vi "SelectCycle.vi"   [LabVIEW 2019]
uses:
  02 Mode/SerialMode/SerialClass.lvclass
  02 Mode/TCPClientMode/TCPClientClass.lvclass
  02 Mode/TCPServerMode/TCPServerClass.lvclass
panel:
  # "带有发送的功能不能和单侦听的挤在一个循环内\n否则会导致时间强行同步，未选中的也要等待发送侦听完成\n\n且对于串口自发自收的情况，由于强制循环同步导致发送方无法准确获取反馈\n因为反馈方在等待状态，完成后才能收到命令再反馈，但是发送方已超时"
types:
  T1 = cluster{"串口名":string, "串口类":refnum<class "SerialClass.lvclass">}
  T2 = typedef "串口枚举.ctl" = enum16{"ini", "增", "删", "查", "改"}
  T3 = cluster{"客服名":string, "客服类":refnum<class "TCPClientClass.lvclass">}
  T4 = cluster{"没有记录？":bool, "串口类":refnum<class "SerialClass.lvclass">}
  T5 = typedef "SerialData.ctl" = cluster{"VISA串口名称":refnum<visa-resource-name>, "波特率":u32, "停止位":u16, "流控制":u16, "数据位":u16, "奇偶校验":enum16{"None", "Odd", "Even", "Mark", "Space"}, "超时":u32, "启用终止符？":bool, "终止符":u8}
  T6 = cluster{"未找到?":bool, "客服类":refnum<class "TCPClientClass.lvclass">}
  T7 = map{string, refnum<class "TCPServerClass.lvclass">}
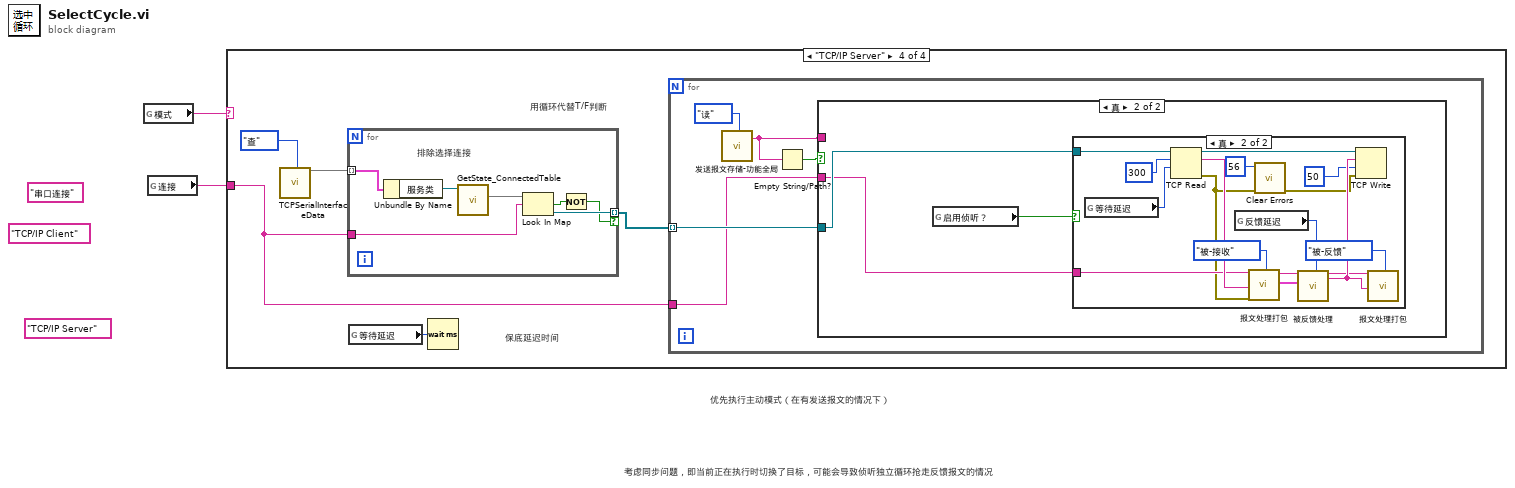
[diagram p0: block diagram]
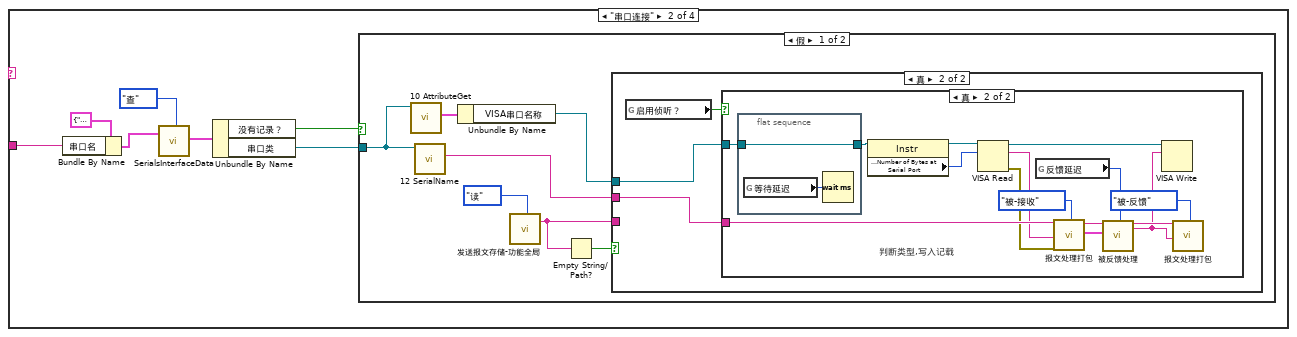
[diagram p3: hidden frame]
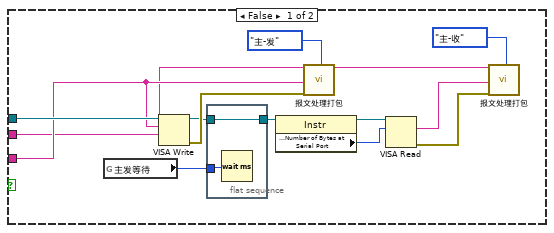
[diagram p4: hidden frame]
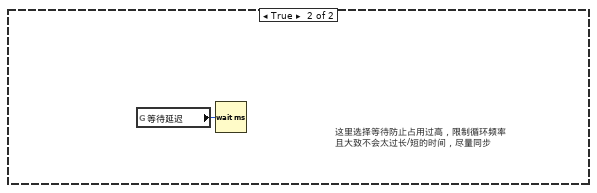
[diagram p6: hidden frame]
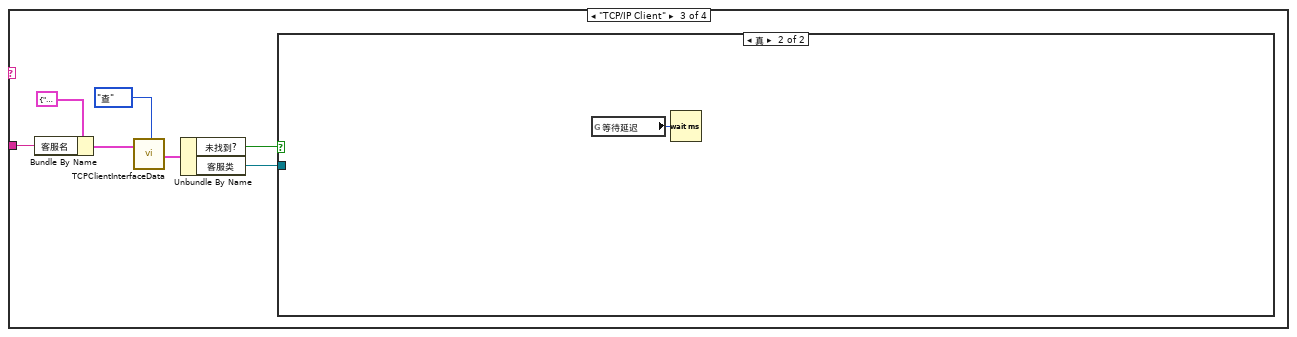
[diagram p7: hidden frame]
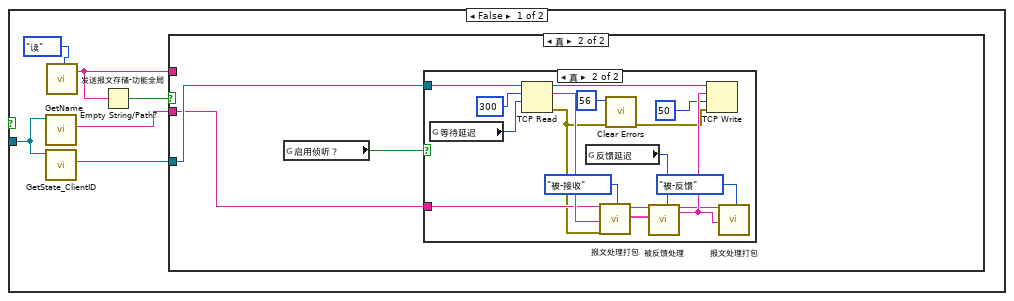
[diagram p8: hidden frame]
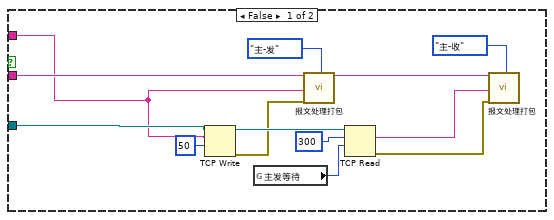
[diagram p9: hidden frame]
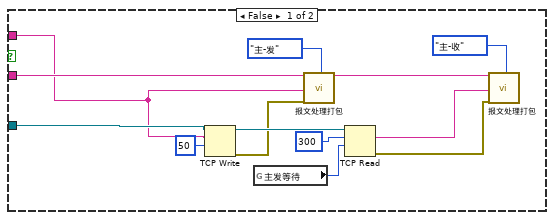
[diagram p11: hidden frame]
diagram:
  (unwired) "TCP/IP Server" ("y")
  (unwired) "TCP/IP Client" ("y")
  (unwired) "串口连接" ("y")
  # "考虑同步问题，即当前正在执行时切换了目标，可能会导致侦听独立循环抢走反馈报文的情况"
  # "优先执行主动模式（在有发送报文的情况下）"
  n1 = global read "全局-配置识别.vi" "模式"() -> (w2:string)
  n2 = global read "全局-配置识别.vi" "连接"() -> (w1:string)
  n3 = case shown="\"TCP/IP Server\"" w2 {
    tunnel: w1 -> [_ w3 w59 w102]
    frame "假", Default {
    }
    frame "串口连接" {
      n4 = Bundle By Name(cluster=T1 {"串口名"="", "串口类"=refnum} ("信息"), "串口名"=w3) -> (w7:T1)
      n5 = call "SerialsInterfaceData.vi"("信息"=w7, "串口枚举"=串口枚举."查") -> ("查找结果"=w6:T4)  [unwired: 16 in, 1 out]
      n6 = Unbundle By Name(w6) -> ("没有记录？"=w5:bool, "串口类"=w4:refnum<class "SerialClass.lvclass">)
      n7 = case shown="假" w5 {
        tunnel: w4 -> [w15 _]
        frame False {
          n8 = call-dynamic "10 AttributeGet.vi"("SerialClass 输入"=w15) -> ("串口配置"=w16:T5)  [unwired: 7 in, 3 out]
          n9 = call-dynamic "12 SerialName.vi"("SerialClass 输入"=w15) -> ("串口名称"=w11:string)  [unwired: 8 in, 2 out]
          n10 = Unbundle By Name(w16) -> ("VISA串口名称"=w10:refnum<visa-resource-name>)
          n11 = call "发送报文存储-功能全局.vi"("枚举"=enum16{"ini", "读", "写"}."读") -> ("报文输出"=w14:string)  [unwired: 18 in]
          n12 = Empty String/Path?(string/path=w14) -> (empty?=w13:bool)
          n13 = case shown="真" w13 {
            tunnel: w10 -> [w28 w34]
            tunnel: w14 -> [w23 _]
            tunnel: w11 -> [w17 w33]
            frame False {
              n14 = global read "全局-配置识别.vi" "主发等待"() -> (w18:u32)
              n15 = VISA Write(VISA resource name=w28, write buffer=w23) -> (VISA resource name out=w20:refnum<visa-resource-name>, error out=w21:errorcluster)  [unwired: 1 in, 1 out]
              n16 = flat-sequence {
                tunnel: w20 -> [w32]
                tunnel: [w32] -> w19
                tunnel: w18 -> [w31]
                frame #0 {
                  n17 = Wait (ms)(milliseconds to wait=w31) -> ()  [unwired: 1 out]
                }
              }
              n18 = property class="Instr"(reference=w19) -> (reference out=w29:refnum<visa-resource-name>, "Serial Settings:Number of Bytes at Serial Port"=w30:u32)  [unwired: 1 in, 1 out]
              n19 = call "报文处理打包.vi"("识别名称"=w17, "报文"=w23, "Error In"=w21, "类型"=enum16{"被-接收", "被-反馈", "主-发", "主-收"}."主-发") -> ("识别名称输出"=w24:string)  [unwired: 14 in, 1 out]
              n20 = VISA Read(VISA resource name=w29, byte count=w30) -> (read buffer=w25:string, error out=w22:errorcluster)  [unwired: 1 in, 2 out]
              n21 = call "报文处理打包.vi"("识别名称"=w24, "报文"=w25, "Error In"=w22, "类型"=enum16{"被-接收", "被-反馈", "主-发", "主-收"}."主-收") -> ()  [unwired: 14 in, 2 out]
            }
            frame True {
              n22 = global read "全局-被反馈配置.vi" "启用侦听？"() -> (w35:bool)
              n23 = case shown="真" w35 {
                tunnel: w34 -> [_ w36]
                tunnel: w33 -> [_ w48]
                frame False {
                }
                frame True {
                  # "判断类型,写入记载"
                  n24 = flat-sequence {
                    tunnel: [w52] -> w37
                    tunnel: w36 -> [w52]
                    frame #0 {
                      n25 = global read "全局-配置识别.vi" "等待延迟"() -> (w51:u32)
                      n26 = Wait (ms)(milliseconds to wait=w51) -> ()  [unwired: 1 out]
                    }
                  }
                  n27 = property class="Instr"(reference=w37) -> (reference out=w50:refnum<visa-resource-name>, "Serial Settings:Number of Bytes at Serial Port"=w49:u32)  [unwired: 1 in, 1 out]
                  n28 = VISA Read(VISA resource name=w50, byte count=w49) -> (VISA resource name out=w45:refnum<visa-resource-name>, read buffer=w47:string, error out=w44:errorcluster)  [unwired: 1 in, 1 out]
                  n29 = global read "全局-配置识别.vi" "反馈延迟"() -> (w38:u32)
                  n30 = call "报文处理打包.vi"("识别名称"=w48, "报文"=w47, "Error In"=w44, "类型"=enum16{"被-接收", "被-反馈", "主-发", "主-收"}."被-接收") -> ("识别名称输出"=w43:string, "被收校验信息"=w42:cluster{"可用？":bool, "功能码":u8, "无crc报文":u8[]})  [unwired: 14 in]
                  n31 = call "被反馈处理.vi"("识别名称"=w43, "校验信息"=w42, "等待时间（毫秒）"=w38) -> ("识别名称输出"=w41:string, "反馈"=w40:string)  [unwired: 15 in]
                  n32 = VISA Write(VISA resource name=w45, write buffer=w40) -> ()  [unwired: 1 in, 3 out]
                  n33 = call "报文处理打包.vi"("识别名称"=w41, "报文"=w40, "类型"=enum16{"被-接收", "被-反馈", "主-发", "主-收"}."被-反馈") -> ()  [unwired: 15 in, 2 out]
                }
              }
            }
          }
        }
        frame True {
          # "这里选择等待防止占用过高，限制循环频率\n且大致不会太过长/短的时间，尽量同步"
          n34 = global read "全局-配置识别.vi" "等待延迟"() -> (w53:u32)
          n35 = Wait (ms)(milliseconds to wait=w53) -> ()  [unwired: 1 out]
        }
      }
    }
    frame "TCP/IP Client" {
      n36 = Bundle By Name(cluster=T3 {"客服名"="", "客服类"=refnum} ("信息"), "客服名"=w59) -> (w58:T3)
      n37 = call "TCPClientInterfaceData.vi"("信息"=w58, "客服接口枚举"=enum16{"ini", "增", "删", "查", "改"}."查") -> ("查找结果"=w56:T6)  [unwired: 16 in, 1 out]
      n38 = Unbundle By Name(w56) -> ("未找到?"=w55:bool, "客服类"=w54:refnum<class "TCPClientClass.lvclass">)
      n39 = case shown="真" w55 {
        tunnel: w54 -> [w62 _]
        frame False {
          n40 = call-dynamic "GetName.vi"("TCPClientClass 输入"=w62) -> ("结果字符串"=w61:string)  [unwired: 8 in, 2 out]
          n41 = call-dynamic "GetState_ClientID.vi"("TCPClientClass输入"=w62) -> ("连接ID"=w63:refnum<k5>)  [unwired: 8 in, 2 out]
          n42 = call "发送报文存储-功能全局.vi"("枚举"=enum16{"ini", "读", "写"}."读") -> ("报文输出"=w66:string)  [unwired: 18 in]
          n43 = Empty String/Path?(string/path=w66) -> (empty?=w65:bool)
          n44 = case shown="真" w65 {
            tunnel: w63 -> [w79 w81]
            tunnel: w66 -> [w74 _]
            tunnel: w61 -> [w75 w80]
            frame False {
              n45 = TCP Write(connection ID=w79, data in=w74, 9:50 ("超时毫秒(25000)")) -> (connection ID out=w72:refnum<k5>, error out=w71:errorcluster)  [unwired: 1 in, 1 out]
              n46 = global read "全局-配置识别.vi" "主发等待"() -> (w70:u32)
              n47 = call "报文处理打包.vi"("识别名称"=w75, "报文"=w74, "Error In"=w71, "类型"=enum16{"被-接收", "被-反馈", "主-发", "主-收"}."主-发") -> ("识别名称输出"=w76:string)  [unwired: 14 in, 1 out]
              n48 = TCP Read(connection ID=w72, bytes to read=300 ("读取的字节"), 9:w70) -> (data out=w67:string, error out=w68:errorcluster)  [unwired: 2 in, 1 out]
              n49 = call "报文处理打包.vi"("识别名称"=w76, "报文"=w67, "Error In"=w68, "类型"=enum16{"被-接收", "被-反馈", "主-发", "主-收"}."主-收") -> ()  [unwired: 14 in, 2 out]
            }
            frame True {
              n50 = global read "全局-被反馈配置.vi" "启用侦听？"() -> (w82:bool)
              n51 = case shown="真" w82 {
                tunnel: w81 -> [_ w99]
                tunnel: w80 -> [_ w93]
                frame False {
                }
                frame True {
                  n52 = global read "全局-配置识别.vi" "等待延迟"() -> (w98:u32)
                  n53 = TCP Read(connection ID=w99, bytes to read=300 ("读取的字节"), 9:w98) -> (connection ID out=w83:refnum<k5>, data out=w95:string, error out=w86:errorcluster)  [unwired: 2 in]
                  n54 = global read "全局-配置识别.vi" "反馈延迟"() -> (w87:u32)
                  n55 = call "报文处理打包.vi"("识别名称"=w93, "报文"=w95, "Error In"=w86, "类型"=enum16{"被-接收", "被-反馈", "主-发", "主-收"}."被-接收") -> ("识别名称输出"=w91:string, "被收校验信息"=w90:cluster{"可用？":bool, "功能码":u8, "无crc报文":u8[]})  [unwired: 14 in]
                  n56 = call <vilib>:"Clear Errors.vi"("error in (no error)"=w86, "specific error code to clear (0: all)"=56) -> ("error out"=w84:errorcluster)  [unwired: 4 in, 1 out]
                  n57 = call "被反馈处理.vi"("识别名称"=w91, "校验信息"=w90, "等待时间（毫秒）"=w87) -> ("识别名称输出"=w89:string, "反馈"=w96:string)  [unwired: 15 in]
                  n58 = TCP Write(connection ID=w83, data in=w96, error in (no error)=w84, 9:50 ("超时毫秒(25000)")) -> ()  [unwired: 3 out]
                  n59 = call "报文处理打包.vi"("识别名称"=w89, "报文"=w96, "类型"=enum16{"被-接收", "被-反馈", "主-发", "主-收"}."被-反馈") -> ()  [unwired: 15 in, 2 out]
                }
              }
            }
          }
        }
        frame True {
          n60 = global read "全局-配置识别.vi" "等待延迟"() -> (w100:u32)
          n61 = Wait (ms)(milliseconds to wait=w100) -> ()  [unwired: 1 out]
        }
      }
    }
    frame "TCP/IP Server" {
      # "用循环代替T/F判断"
      # "保底延迟时间"
      n62 = call "TCPSerialInterfaceData.vi"("客服接口枚举"=enum16{"ini", "增", "删", "查", "改", "腾笼换鸟"}."查") -> ("服务表"=w105:T7)  [unwired: 17 in, 1 out]
      n63 = for {
        tunnel: w105 -> [w150] mode=indexing
        tunnel: [w147] -> w103 mode=indexing if=w145
        tunnel: w102 -> [w144]
        # "排除选择连接"
        n64 = Unbundle By Name(w150) -> ("服务类"=w149:refnum<class "TCPServerClass.lvclass">)
        n65 = call-dynamic "GetState_ConnectedTable.vi"("TCPServerClass输入"=w149) -> ("连接端ID表"=w148:map{string, refnum<k5>})  [unwired: 8 in, 2 out]
        n66 = Look In Map(map=w148, key=w144) -> (key not found?=w146:bool, value=w147:refnum<k5>)  [unwired: 1 in]
        n67 = Not(x=w146) -> (.not. x?=w145:bool)
      }
      n68 = global read "全局-配置识别.vi" "等待延迟"() -> (w101:u32)
      n69 = Wait (ms)(milliseconds to wait=w101) -> ()  [unwired: 1 out]
      n70 = for {
        tunnel: w103 -> [w107] mode=indexing
        tunnel: w102 -> [w106]
        n71 = call "发送报文存储-功能全局.vi"("枚举"=enum16{"ini", "读", "写"}."读") -> ("报文输出"=w109:string)  [unwired: 18 in]
        n72 = Empty String/Path?(string/path=w109) -> (empty?=w110:bool)
        n73 = case shown="真" w110 {
          tunnel: w107 -> [w123 w125]
          tunnel: w109 -> [w118 _]
          tunnel: w106 -> [w119 w124]
          frame False {
            n74 = TCP Write(connection ID=w123, data in=w118, 9:50 ("超时毫秒(25000)")) -> (connection ID out=w116:refnum<k5>, error out=w115:errorcluster)  [unwired: 1 in, 1 out]
            n75 = global read "全局-配置识别.vi" "主发等待"() -> (w114:u32)
            n76 = call "报文处理打包.vi"("识别名称"=w119, "报文"=w118, "Error In"=w115, "类型"=enum16{"被-接收", "被-反馈", "主-发", "主-收"}."主-发") -> ("识别名称输出"=w120:string)  [unwired: 14 in, 1 out]
            n77 = TCP Read(connection ID=w116, bytes to read=300 ("读取的字节"), 9:w114) -> (data out=w111:string, error out=w112:errorcluster)  [unwired: 2 in, 1 out]
            n78 = call "报文处理打包.vi"("识别名称"=w120, "报文"=w111, "Error In"=w112, "类型"=enum16{"被-接收", "被-反馈", "主-发", "主-收"}."主-收") -> ()  [unwired: 14 in, 2 out]
          }
          frame True {
            n79 = global read "全局-被反馈配置.vi" "启用侦听？"() -> (w126:bool)
            n80 = case shown="真" w126 {
              tunnel: w125 -> [_ w143]
              tunnel: w124 -> [_ w137]
              frame False {
              }
              frame True {
                n81 = global read "全局-配置识别.vi" "等待延迟"() -> (w142:u32)
                n82 = TCP Read(connection ID=w143, bytes to read=300 ("读取的字节"), 9:w142) -> (connection ID out=w127:refnum<k5>, data out=w139:string, error out=w130:errorcluster)  [unwired: 2 in]
                n83 = global read "全局-配置识别.vi" "反馈延迟"() -> (w131:u32)
                n84 = call "报文处理打包.vi"("识别名称"=w137, "报文"=w139, "Error In"=w130, "类型"=enum16{"被-接收", "被-反馈", "主-发", "主-收"}."被-接收") -> ("识别名称输出"=w135:string, "被收校验信息"=w134:cluster{"可用？":bool, "功能码":u8, "无crc报文":u8[]})  [unwired: 14 in]
                n85 = call <vilib>:"Clear Errors.vi"("error in (no error)"=w130, "specific error code to clear (0: all)"=56) -> ("error out"=w128:errorcluster)  [unwired: 4 in, 1 out]
                n86 = call "被反馈处理.vi"("识别名称"=w135, "校验信息"=w134, "等待时间（毫秒）"=w131) -> ("识别名称输出"=w133:string, "反馈"=w140:string)  [unwired: 15 in]
                n87 = TCP Write(connection ID=w127, data in=w140, error in (no error)=w128, 9:50 ("超时毫秒(25000)")) -> ()  [unwired: 3 out]
                n88 = call "报文处理打包.vi"("识别名称"=w133, "报文"=w140, "类型"=enum16{"被-接收", "被-反馈", "主-发", "主-收"}."被-反馈") -> ()  [unwired: 15 in, 2 out]
              }
            }
          }
        }
      }
    }
  }
